vi "Elevator Bang Bang.vi"(6 "Totes Mode":bool, 7 "Number Totes":dbl, 8 "Hold Up Mode":bool, 9 "Top":bool, 10 "Middle":bool, 11 "Bottom":bool) -> (3 "in range":bool)   [LabVIEW 2014]
uses:
  Robot Global Data.vi
panel:
  out "Pot Value":dbl
  in  "Last Fed Value":dbl
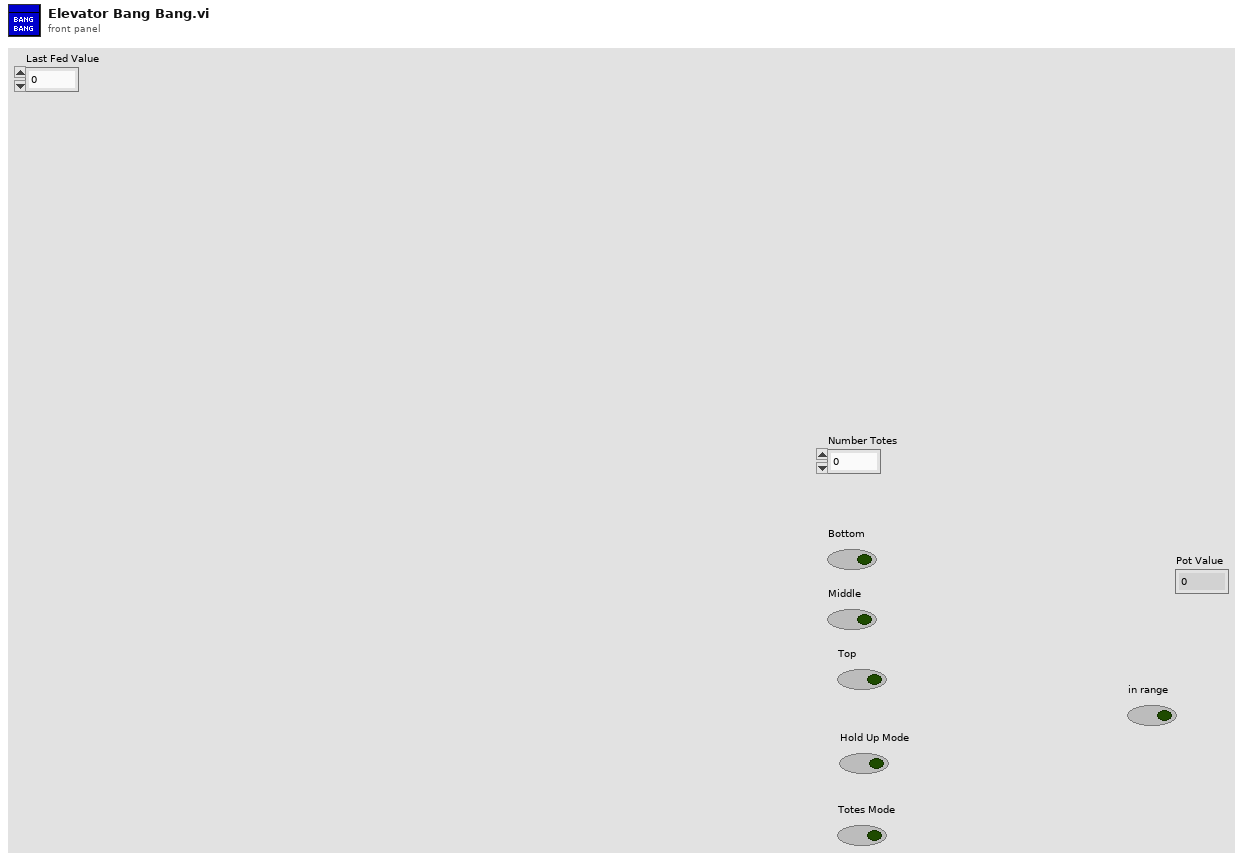
[diagram p1: front panel]
types:
  T1 = typedef "WPI_PotentiometerDevRef.ctl" = cluster{"DevStatus":errorcluster, "Controller":T2, "Analog Channel":T3, "Invert Output":bool}
  T2 = typedef "FPGA_TypedefAnalogModule.ctl" = enum16{"Controller 1"}
  T3 = typedef "FPGA_AIChannel.ctl" = enum8{"AI 0", "AI 1", "AI 2", "AI 3", "AI MXP 0", "AI MXP 1", "AI MXP 2", "AI MXP 3", "Invalid"}
  T4 = typedef "WPI_MotorControlDeviceRef.ctl" = cluster{"DeviceStatus":errorcluster, "Type":T5, "PWM":cluster{"Controller":T6, "PWM Channel":T7, "DeadBand":T8}, "CAN":cluster{"Device Number":u8, "Control Mode":T9, "Semaphore":T10, "Max Vout":dbl, "TalonSRX Control Mode":T11}, "Invert":bool, "TransformRef":T12, "InvTransformRef":T12}
  T5 = typedef "WPI_MotorControlType.ctl" = enum16{"PWM", "CAN", "CANTalonSRX"}
  T6 = typedef "FPGA_TypedefDigitalModule.ctl" = enum16{"Controller 1"}
  T7 = typedef "FPGA_DIOPWMChannel.ctl" = enum8{"PWM 0", "PWM 1", "PWM 2", "PWM 3", "PWM 4", "PWM 5", "PWM 6", "PWM 7", "PWM 8", "PWM 9", "PWM MXP 0", "PWM MXP 1", "PWM MXP 2", "PWM MXP 3", "PWM MXP 4", "PWM MXP 5", "PWM MXP 6", "PWM MXP 7", "PWM MXP 8", "PWM MXP 9", "Invalid"}
  T8 = typedef "WPI_PWMDeadband.ctl" = cluster{"Name":string, "maxPositivePwm":i32, "minPositivePwm":i32, "centerPwm":i32, "maxNegativePwm":i32, "minNegativePwm":i32, "angularRange":u16}
  T9 = typedef "WPI_CANJaguar_ControlMode.ctl" = enum8{"Percent VBus", "Current", "Speed", "Position", "Voltage"}
  T10 = typedef "Semaphore RefNum" = refnum<k1>
  T11 = typedef "WPI_CANTalonSRX_APIControlMode.ctl" = enum8{"Percent VBus", "Speed", "Position", "Slave", "Unchanged / Invalid"}
  T12 = typedef "WPI_PWMTransform_ConPane.ctl" = refnum<vi>
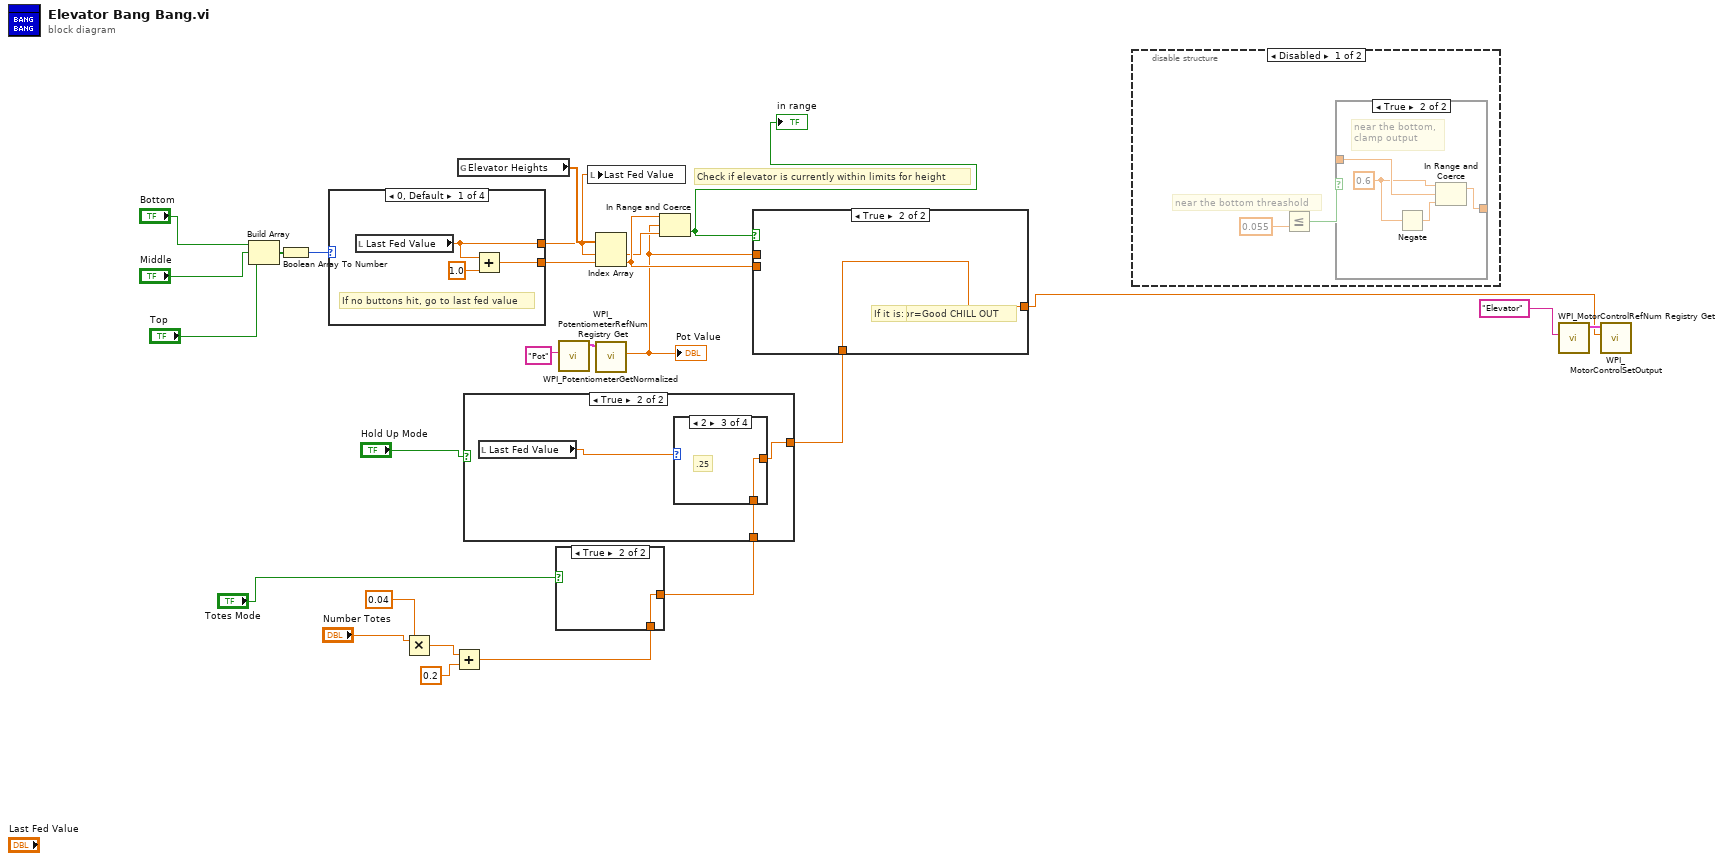
[diagram p0: block diagram]
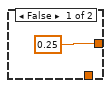
[diagram p4: hidden frame]
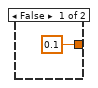
[diagram p5: hidden frame]
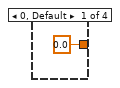
[diagram p6: hidden frame]
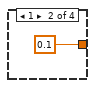
[diagram p7: hidden frame]
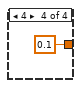
[diagram p8: hidden frame]
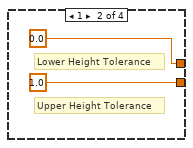
[diagram p9: hidden frame]
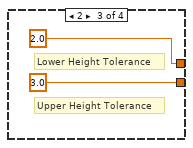
[diagram p10: hidden frame]
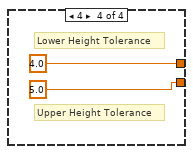
[diagram p11: hidden frame]
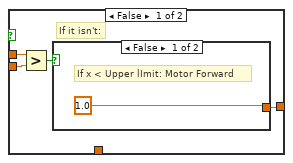
[diagram p12: hidden frame]
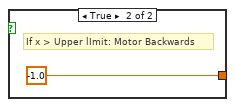
[diagram p13: hidden frame]
diagram:
  # "Check if elevator is currently within limits for height"
  n1 = Build Array("Bottom", "Middle", "Top") -> (w21:bool[])
  n2 = Boolean Array To Number(Boolean array=w21) -> (number=w12:u32)
  n3 = case shown="0, Default" w12 {
    tunnel: [w29 0.0 ("element") 2.0 ("element") 4.0 ("element")] -> w20
    tunnel: [w27 1.0 ("element") 3.0 ("element") 5.0 ("element")] -> w22
    frame 0, Default {
      # "If no buttons hit, go to last fed value"
      n4 = local read "Last Fed Value"() -> (w29:dbl)
      n5 = Add(x=w29, y=1.0) -> (x+y=w27:dbl)
    }
    frame 1 {
      # "Upper Height Tolerance"
      # "Lower Height Tolerance"
    }
    frame 2 {
      # "Upper Height Tolerance"
      # "Lower Height Tolerance"
    }
    frame 4 {
      # "Upper Height Tolerance"
      # "Lower Height Tolerance"
    }
  }
  n6 = Multiply(x="Number Totes", y=0.04) -> (x*y=w4:dbl)
  n7 = Add(x=w4, y=0.2) -> (x+y=w3:dbl)
  n8 = global read "Robot Global Data.vi" "Elevator Heights"() -> (w23:dbl[])
  n9 = case shown="True" "Totes Mode" {
    tunnel: [0.25 ("Output") w37] -> w6
    tunnel: w3 -> [_ w37]
    frame False {
    }
    frame True {
    }
  }
  n10 = case shown="True" "Hold Up Mode" {
    tunnel: [0.1 ("Output") w41] -> w13
    tunnel: w6 -> [_ w39]
    frame False {
    }
    frame True {
      n11 = local read "Last Fed Value"() -> (w40:dbl)
      n12 = case shown="2" w40 {
        tunnel: [0.0 ("Output") 0.1 ("Output") w44 0.1 ("Output")] -> w41
        tunnel: w39 -> [_ _ w44 _]
        frame 0, Default {
        }
        frame 1 {
        }
        frame 2 {
          # ".25"
        }
        frame 4 {
        }
      }
    }
  }
  n13 = call <vilib>:"WPI_PotentiometerRefNum Registry Get.vi"("refnum name"="Pot") -> ("PotDevRef"=w26:T1)  [unwired: 9 in, 1 out]
  n14 = local write "Last Fed Value"(w20) -> ()
  n15 = Index Array(array=w23, index #1=w20, index #2=w22) -> (element #1=w14:dbl, element #2=w15:dbl)
  n16 = call <vilib>:"WPI_PotentiometerGetNormalized.vi"("PotDevRef"=w26) -> ("Normalized Value"=w9:dbl)  [unwired: 8 in, 2 out]
  "Pot Value" <- w9
  n17 = In Range and Coerce(upper limit=w15, x=w9, lower limit=w14) -> (In Range?=w16:bool)  [unwired: 1 out]
  "in range" <- w16
  n18 = case shown="True" w16 {
    tunnel: w9 -> [w48 _]
    tunnel: w15 -> [w47 _]
    tunnel: w13 -> [_ w52]
    tunnel: [w46 w52] -> w1
    frame False {
      # "If it isn't:"
      n19 = Greater?(x=w48, y=w47) -> (0:w49:bool)
      n20 = case shown="False" w49 {
        tunnel: [1.0 ("Output") -1.0 ("Output")] -> w46
        frame False {
          # "If x < Upper lImit: Motor Forward"
        }
        frame True {
          # "If x > Upper lImit: Motor Backwards"
        }
      }
    }
    frame True {
      # "If it is:"
      # "Elevator=Good CHILL OUT"
    }
  }
  n21 = disable-structure shown="Disabled" {
    frame Disabled {
      # "near the bottom threashold"
      n22 = Less Or Equal?(y=0.055) -> (x <= y?=w53:bool)  [unwired: 1 in]
      n23 = case shown="True" w53 {
        tunnel: [w55 w59] -> _
        tunnel: _ -> [w55 w58]
        frame False {
          # "not near the bottom"
        }
        frame True {
          w56 = 0.6
          # "near the bottom,\nclamp output"
          n24 = Negate(x=w56) -> (-x=w57:dbl)
          n25 = In Range and Coerce(upper limit=w56, x=w58, lower limit=w57) -> (coerced(x)=w59:dbl)  [unwired: 1 out]
        }
      }
    }
    frame Enabled {
    }
  }
  n26 = call <vilib>:"WPI_MotorControlRefNum Registry Get.vi"("refnum name"="Elevator") -> ("MotorControlDevRef"=w10:T4)  [unwired: 9 in, 1 out]
  n27 = call <vilib>:"WPI_MotorControlSetOutput.vi"("Output"=w1, "MotorControlDevRef"=w10) -> ()  [unwired: 7 in, 3 out]
